vi "Call Functional Global Variable.vi"() -> ()   [LabVIEW 2019]
doc: "This main VI demonstrates a simple usage of a Functional Global Variable to increment and display a number"
uses:
  Resources/Action Items.ctl
panel:
  in  "Increment":bool
  in  "Initialize":bool
  in  "Get":bool
  in  "stop":bool
  out "Result":i32
  in  "Initialize to":i32
  # "Overview: This VI demonstrates a simple usage of a Functional Global Variable to increment and display a number\nRequirements: LabVIEW 2012 (or compatible)\nInstructions:\n1. Run the VI\n2. Set the Initial value of the number and click on Initialize\n3. Click on Increment\n4. Click on Get\n5. Stop Execution"
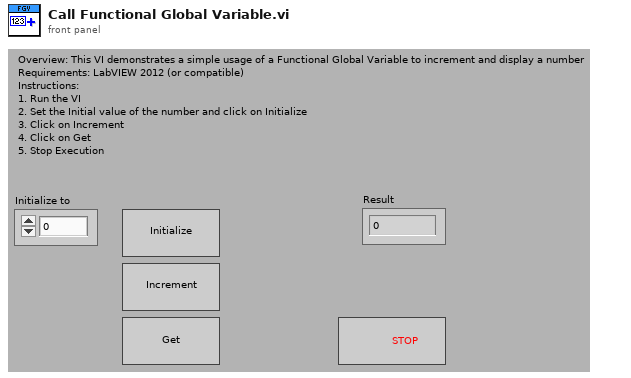
[diagram p1: front panel]
types:
  T1 = typedef "Action Items.ctl" = enum16{"Initialize", "Get", "Increment"}
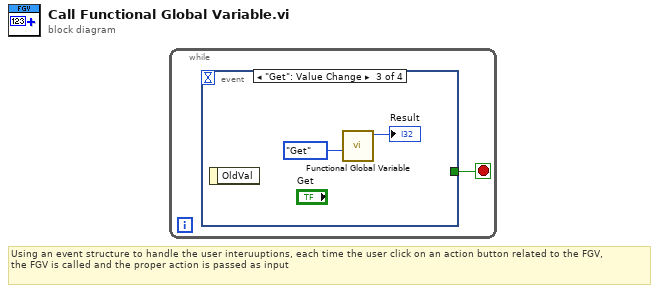
[diagram p0: block diagram]
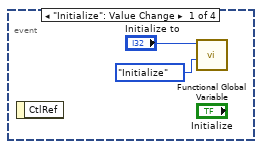
[diagram p2: hidden frame]
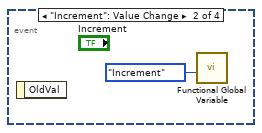
[diagram p3: hidden frame]
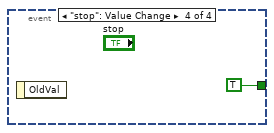
[diagram p4: hidden frame]
diagram:
  # "Using an event structure to handle the user interuuptions, each time the user click on an action button related to the FGV,\nthe FGV is called and the proper action is passed as input"
  n1 = while {
    stop <- w1 stop-if-true
    n2 = event shown="[2] \"Get\": Value Change" {
      selector: _ -> [_ _ _ _]
      dyn-events: _ -> [_ _ _ _]
      timeout: _ -> [_ _ _ _]
      tunnel: [_ _ _ TRUE] -> w1
      event "Initialize": Value Change {
        n3 = event-data() -> ()  [unwired: 1 in, 1 out]
        n4 = call "Functional Global Variable.vi"("Action"=Action_Items."Initialize", "Initialize to"="Initialize to") -> ()  [unwired: 9 in, 1 out]
      }
      event "Increment": Value Change {
        n5 = event-data() -> ()  [unwired: 1 in, 1 out]
        n6 = call "Functional Global Variable.vi"("Action"=Action_Items."Increment") -> ()  [unwired: 10 in, 1 out]
      }
      event "Get": Value Change {
        n7 = event-data() -> ()  [unwired: 1 in, 1 out]
        n8 = call "Functional Global Variable.vi"("Action"=Action_Items."Get") -> ("Result"=→"Result":i32)  [unwired: 10 in]
      }
      event "stop": Value Change {
        n9 = event-data() -> ()  [unwired: 1 in, 1 out]
      }
    }
  }
